vi "myRIO v1.0 Build MUX Configuration I2C.vi"(11 "Channel":T4) -> (2 "Configuration Bitmask Array":bool[][](array[boolean]), 3 "Channel Reservation List":T1)   [LabVIEW 2021]
uses:
  <vilib>/myRIO/Common/Instrument Driver Framework/myRIO v1.0/I2C/typedefs/I2C Channels Enum.ctl
  <vilib>/myRIO/Common/Instrument Driver Framework/myRIO v1.0/Resource Manager/typedefs/myRIO v1.0 Channel Reservation List.ctl
  <vilib>/myRIO/Common/Instrument Driver Framework/myRIO v1.0/Resource Manager/typedefs/myRIO v1.0 Channel Reservation Info.ctl
  <vilib>/myRIO/Common/Instrument Driver Framework/myRIO v1.0/Resource Manager/typedefs/myRIO v1.0 Connector List.ctl
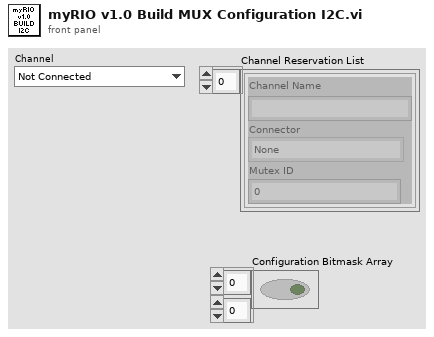
[diagram p1: front panel]
types:
  T1 = typedef "myRIO v1.0 Channel Reservation List.ctl" = T2[]
  T2 = typedef "myRIO v1.0 Channel Reservation Info.ctl" = cluster{"Channel Name":string, "Connector":T3, "Mutex ID":i32}
  T3 = typedef "myRIO v1.0 Connector List.ctl" = enum32{"None", "ConnectorA", "ConnectorB", "ConnectorC"}
  T4 = typedef "I2C Channels Enum.ctl" = enum16{"Not Connected", "A/I2C", "B/I2C", "I2C/I2C"}
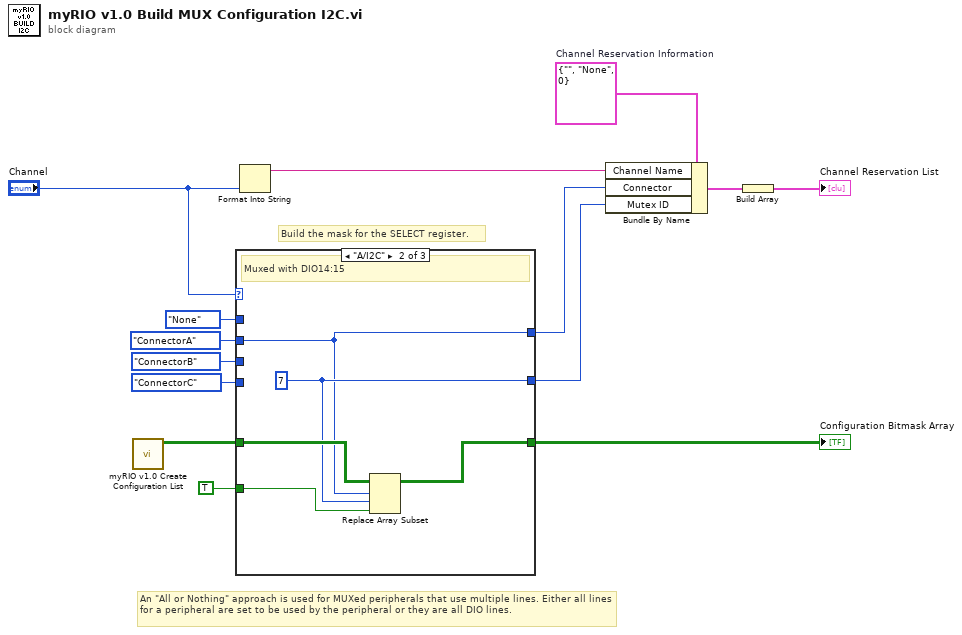
[diagram p0: block diagram]
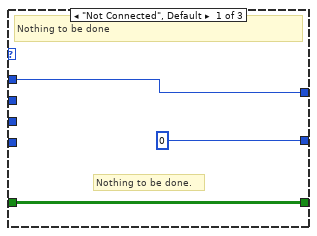
[diagram p2: hidden frame]
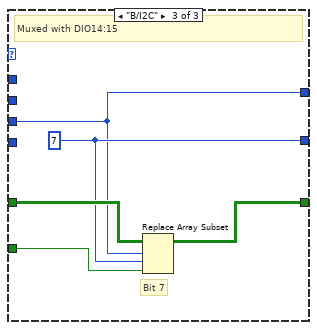
[diagram p3: hidden frame]
diagram:
  w5 = T2 {"Channel Name"="", "Connector"=enum."None", "Mutex ID"=0}  # Channel Reservation Information
  # "An \"All or Nothing\" approach is used for MUXed peripherals that use multiple lines. Either all lines for a peripheral are set to be used by the peripheral or they are all DIO lines."
  # "Build the mask for the SELECT register."
  n1 = call <vilib>:"myRIO v1.0 Create Configuration List.vi"() -> ("Bitmask Array"=w3:bool[][])  [unwired: 11 in]
  n2 = case shown="\"A/I2C\"" "Channel" {
    tunnel: w3 -> [w17 w22 w27]
    tunnel: [w17 w21 w26] -> w11
    tunnel: myRIO_v1.0_Connector_List."None" ("Connector List") -> [w16 _ _]
    tunnel: myRIO_v1.0_Connector_List."ConnectorA" ("Connector List") -> [_ w18 _]
    tunnel: TRUE ("new element/subarray") -> [_ w20 w25]
    tunnel: myRIO_v1.0_Connector_List."ConnectorB" ("Connector List") -> [_ _ w23]
    tunnel: myRIO_v1.0_Connector_List."ConnectorC" ("Connector List") -> [_ _ _]
    tunnel: [0 ("index") w19 w24] -> w7
    tunnel: [w16 w18 w23] -> w8
    frame "Not Connected", Default {
      # "Nothing to be done."
      # "Nothing to be done"
    }
    frame "A/I2C" {
      w19 = 7 ("index")
      # "Muxed with DIO14:15"
      n3 = Replace Array Subset(array=w22, new element=w20, index (row)=w18, index (col)=w19) -> (w21:bool[][])
    }
    frame "B/I2C" {
      w24 = 7 ("index")
      # "Bit 7"
      # "Muxed with DIO14:15"
      n4 = Replace Array Subset(array=w27, new element=w25, index (row)=w23, index (col)=w24) -> (w26:bool[][])
    }
  }
  "Configuration Bitmask Array" <- w11
  n5 = Format Into String("Channel") -> (resulting string=w4:string)  [unwired: 3 in, 1 out]
  n6 = Bundle By Name(cluster=w5, "Channel Name"=w4, "Connector"=w8, "Mutex ID"=w7) -> (w2:T2)
  n7 = Build Array(w2) -> (→"Channel Reservation List":T2[])
